vi "lm35 sıcaklık grafik ölçümü.vi"() -> ()   [LabVIEW 2017]
uses:
  <vilib>/Instr/_visa.llb/VISA Configure Serial Port (Instr).vi
panel:
  out "?":dbl
  in  "Stop Button":bool
  in  "baud rate (9600)":u32=9600
  out "TERMOMETER":dbl(slide) scale=0.0..100.0
  out "Waveform Chart":dbl(graph)
  out "Yüksek":bool
  in  "Yüksek":dbl
  in  "Normal":dbl
  out "Normal":bool
  out "Düşük":bool
  in  "Port COM":refnum<visa-resource-name>
  # "USB Control"
  # "LM35"
  # "SETTINGS"
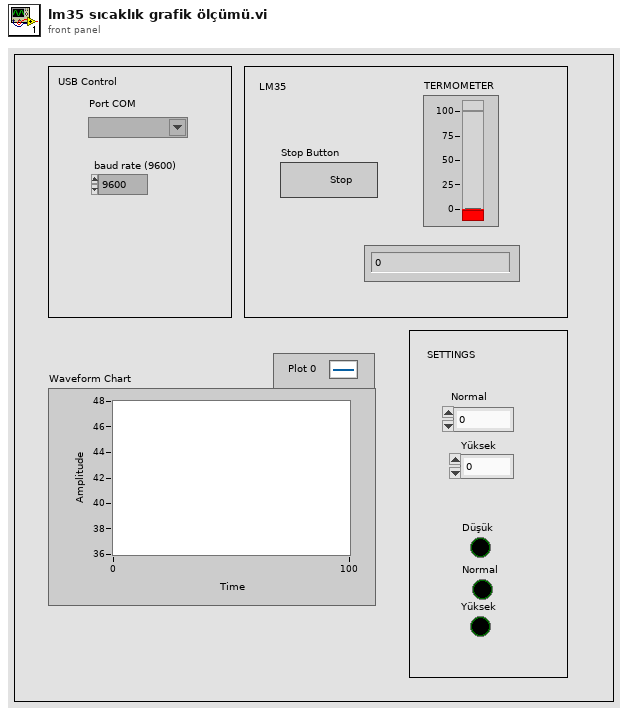
[diagram p1: front panel]
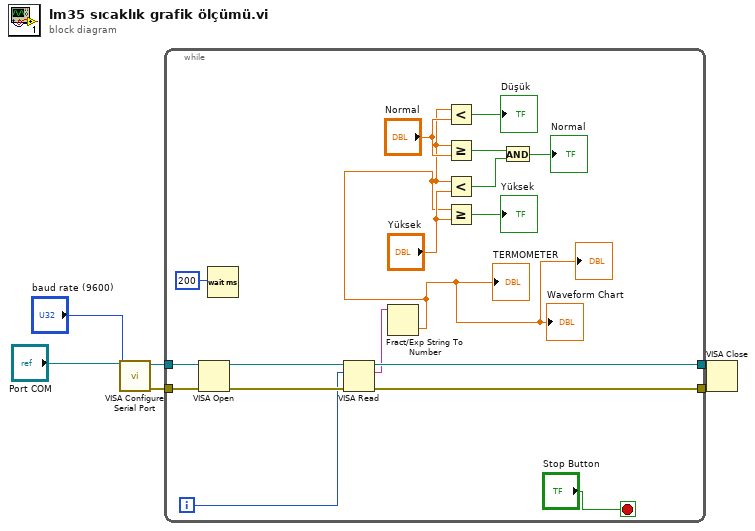
[diagram p0: block diagram]
diagram:
  n1 = call-poly "VISA Configure Serial Port"("VISA resource name"="Port COM", "baud rate (9600)"="baud rate (9600)") -> ("VISA resource name out"=w3:refnum<visa-resource-name>, "error out"=w6:errorcluster)  [unwired: 12 in]
  n2 = while {
    tunnel: w6 -> [w24]
    tunnel: [w22] -> w5
    tunnel: [w21] -> w4
    tunnel: w3 -> [w19]
    i -> [w17]
    stop <- "Stop Button" stop-if-true
    n3 = VISA Open(error in (no error)=w24, VISA resource name=w19) -> (VISA resource name=w20:refnum<visa-resource-name>, error out=w23:errorcluster)  [unwired: 3 in]
    n4 = Wait (ms)(milliseconds to wait=u32 200 ("millisecond timer value")) -> ()  [unwired: 1 out]
    n5 = VISA Read(VISA resource name=w20, byte count=w17, error in (no error)=w23) -> (VISA resource name out=w21:refnum<visa-resource-name>, read buffer=w18:string, error out=w22:errorcluster)  [unwired: 1 out]
    n6 = Fract/Exp String To Number(string=w18) -> (number=w7:dbl)  [unwired: 3 in, 1 out]
    "TERMOMETER" <- w7
    "Waveform Chart" <- w7
    "?" <- w7
    n7 = Less?(x=w7, y="Normal") -> (x < y?=→"Düşük":bool)
    n8 = Greater Or Equal?(x=w7, y="Normal") -> (x >= y?=w13:bool)
    n9 = Less?(x=w7, y="Yüksek") -> (x < y?=w12:bool)
    n10 = Greater Or Equal?(x=w7, y="Yüksek") -> (x >= y?=→"Yüksek":bool)
    n11 = And(x=w13, y=w12) -> (x .and. y?=→"Normal":bool)
  }
  n12 = VISA Close(VISA resource name=w4, error in (no error)=w5) -> ()  [unwired: 1 out]
